vi "EMV Flow Detector.vi"(8 "error in (no error)":errorcluster, 10 "ERD Data":T1, 11 ".NET Refnum in":refnum<k24>) -> (0 "error out":errorcluster, 3 ".NET Refnum out":refnum<k24>)   [LabVIEW 2020]
uses:
  Type Definitions/GEA3 HEWH Mixing Valve.ctl
  Type Definitions/GEA3 HEWH ERD Data.ctl
  C:/TechnologyLab/NI-2010/Drivers/GEA3 Toolkit/GEA3 DLL Source/GeaCommunication.dll
  GEA3 DLL Source/GeaCommunication.dll
panel:
  in  "Detection Slope":dbl=0.5 format="%#_13g"
  out "T6 T7 Flow Dectection":bool
  out "Slope History":dbl[](array[numeric])
  out "Current T6 Temperatures Output":dbl[](array[numeric])=[75.0, 75.0, 75.0, 75.0, 75.0, 75.0, 75.0, 75.0, 75.0, 75.0, 75.0]
  out "Slope Chart T7":dbl(graph)
  out "Current T7 Temperatures":dbl[](array[numeric])
  in  "Abnormal Input Temperature":dbl=80.0
  out "Flow Detect?":bool
  in  "Entry":dbl=11.0
  in  "POLLING_TIME_MS":dbl=1000.0
  in  "FLOW_COUNTER_MAX":dbl=15.0
  in  "STARTING_TEMPERATURE":dbl=140.0
  in  "FLOW_COUNTER_THRESHOLD":dbl=1.0
  in  "T6_OFFSET_FROM_TARGET_INDICATING_FLOW":dbl=3.0
  in  "T7_DELTA_INDICATING_FLOW":dbl=10.0
  in  "T6_DELTA_INDICATING_FLOW":dbl=2.0
  in  "T7_DELTA_FLOW_THRESHOLD":dbl=0.5
  in  "T7 STOP-T6 FLOW -THRESHOLD":dbl=4.0
  out "T6 Flow Dectection":bool
  # "T6 Only"
  # "T7 Only"
  # "T6 and T7"
  # "reading now == 0\nreading in the past == 10"
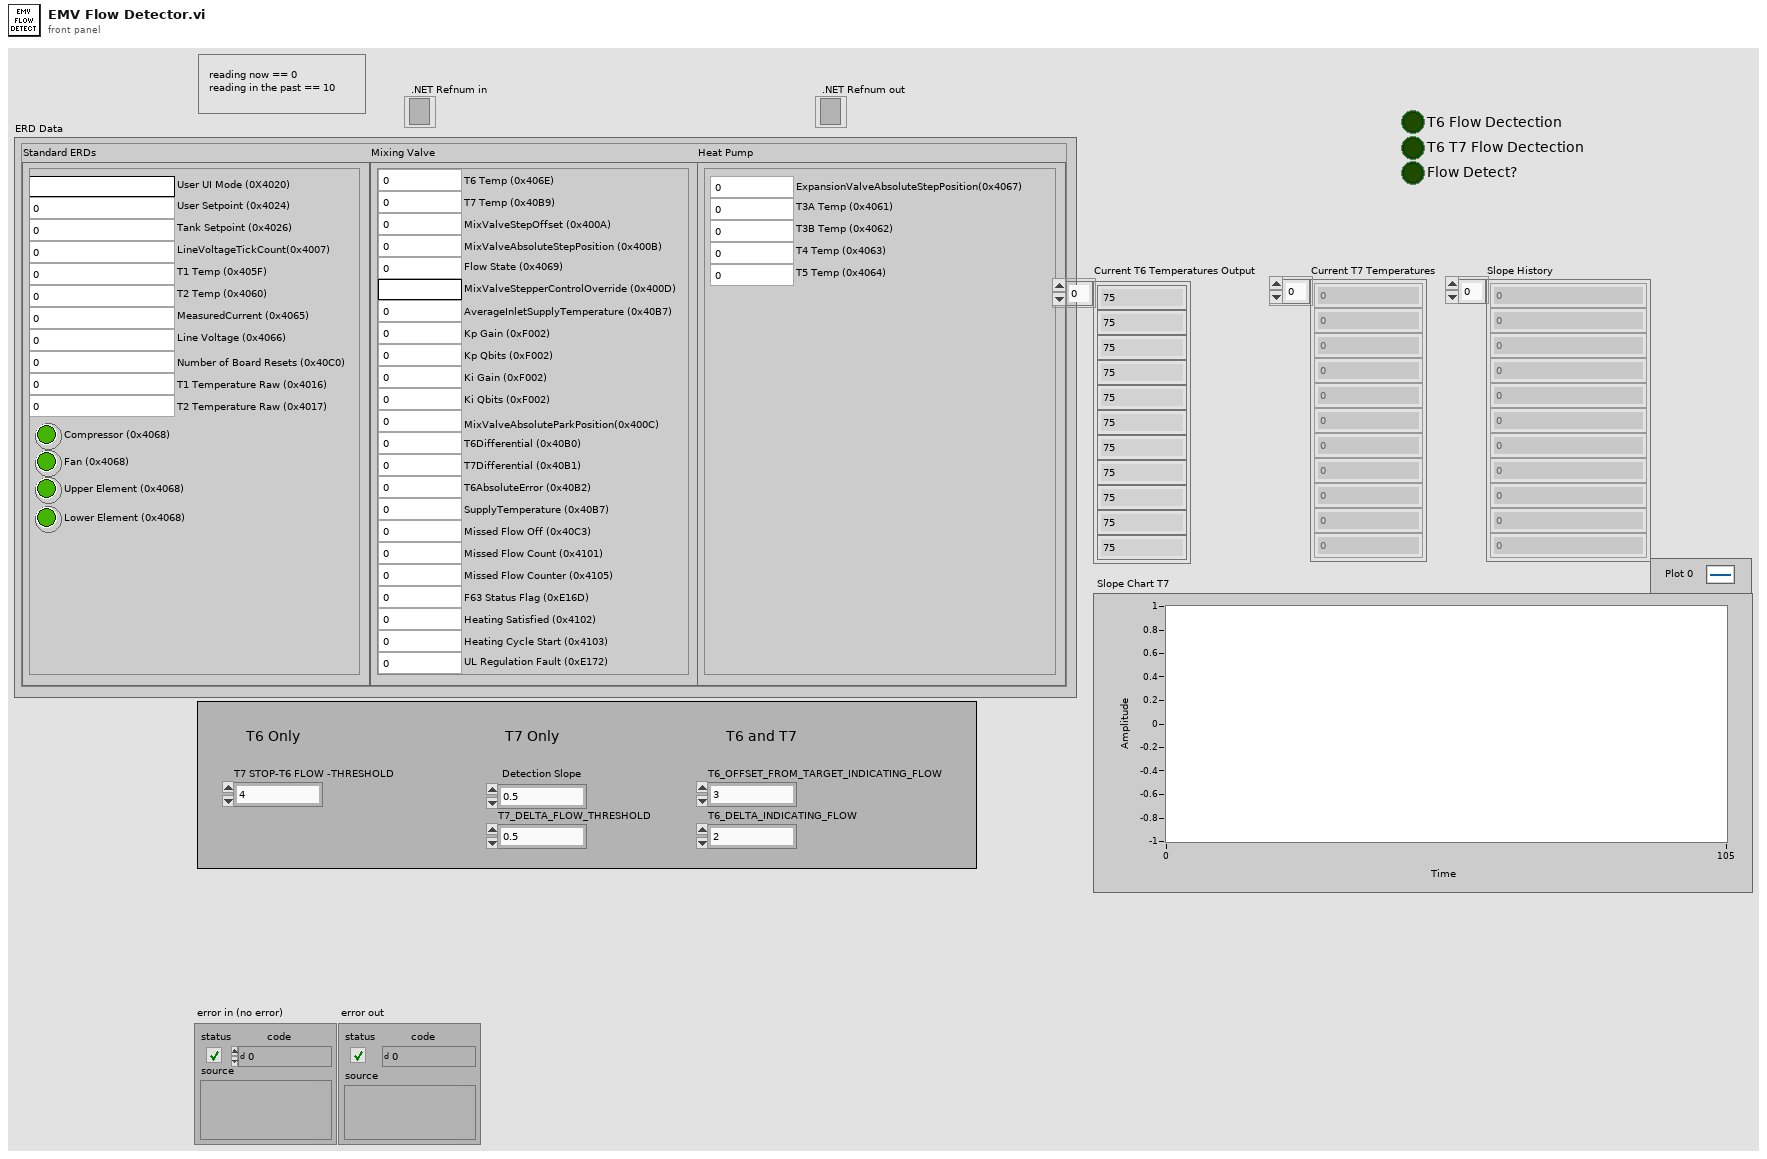
[diagram p1: front panel]
types:
  T1 = typedef "GEA3 HEWH ERD Data.ctl" = cluster{"Mixing Valve":T2, "Standard ERDs":cluster{"User UI Mode (0X4020)":string, "User Setpoint (0x4024)":u16, "Compressor (0x4068)":bool, "Lower Element (0x4068)":bool, "Upper Element (0x4068)":bool, "Fan (0x4068)":bool, "T1 Temp (0x405F)":dbl, "T2 Temp (0x4060)":dbl, "Line Voltage (0x4066)":dbl, "MeasuredCurrent (0x4065)":dbl, "LineVoltageTickCount(0x4007)":u16, "Number of Board Resets (0x40C0)":u16, "T1 Temperature Raw (0x4016)":u16, "T2 Temperature Raw (0x4017)":u16, "Tank Setpoint (0x4026)":u16}, "Heat Pump":cluster{"ExpansionValveAbsoluteStepPosition(0x4067)":i16, "T3A Temp (0x4061)":dbl, "T3B Temp (0x4062)":dbl, "T4 Temp (0x4063)":dbl, "T5 Temp (0x4064)":dbl}}
  T2 = typedef "GEA3 HEWH Mixing Valve.ctl" = cluster{"T7 Temp (0x40B9)":dbl, "MixValveStepOffset (0x400A)":i16, "MixValveAbsoluteStepPosition (0x400B)":i16, "Flow State (0x4069)":u8, "MixValveStepperControlOverride (0x400D)":string, "AverageInletSupplyTemperature (0x40B7)":dbl, "T6 Temp (0x406E)":dbl, "Kp Gain (0xF002)":u16, "Kp Qbits (0xF002)":u16, "Ki Gain (0xF002)":u16, "Ki Qbits (0xF002)":u16, "MixValveAbsoluteParkPosition(0x400C)":i16, "T7Differential (0x40B1)":dbl, "T6Differential (0x40B0)":dbl, "SupplyTemperature (0x40B7)":dbl, "Missed Flow Off (0x40C3)":u8, "T6AbsoluteError (0x40B2)":dbl, "Missed Flow Count (0x4101)":u16, "Missed Flow Counter (0x4105)":u16, "F63 Status Flag (0xE16D)":u16, "Heating Satisfied (0x4102)":u16, "Heating Cycle Start (0x4103)":u16, "UL Regulation Fault (0xE172)":u8}
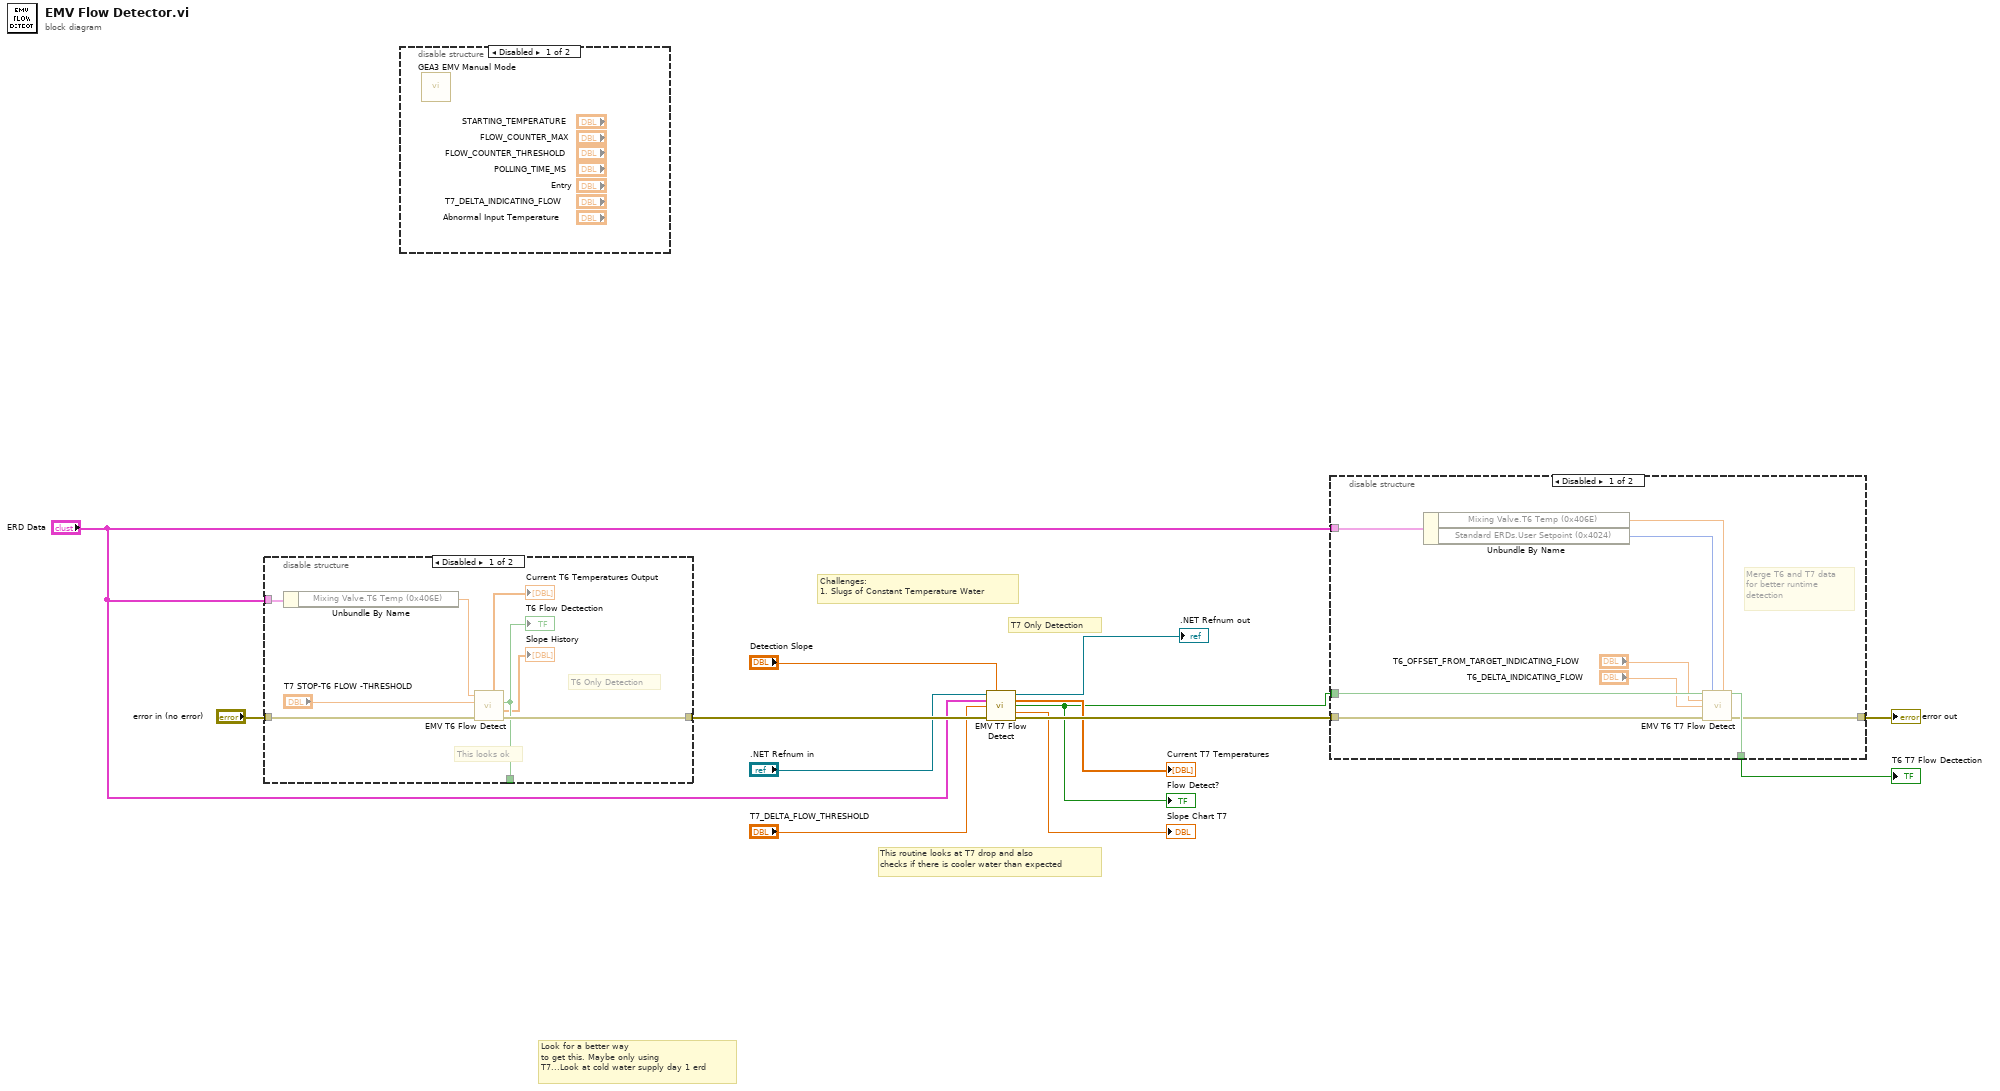
[diagram p0: block diagram]
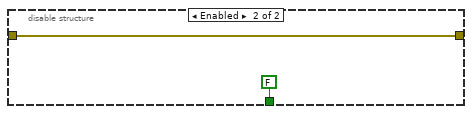
[diagram p4: hidden frame]
diagram:
  # "Challenges:\n1. Slugs of Constant Temperature Water"
  # "T7 Only Detection"
  # "Look for a better way\nto get this. Maybe only using\nT7...Look at cold water supply day 1 erd"
  # "This routine looks at T7 drop and also\nchecks if there is cooler water than expected"
  n1 = disable-structure shown="Disabled" {
    disable-tunnel: "error in (no error)" -> [w21 w23]
    disable-tunnel: [w20 w23] -> w12
    disable-tunnel: [w18 FALSE ("Flow Dectection")] -> _
    disable-tunnel: "ERD Data" -> [w15 _]
    frame Disabled {
      # "T6 Only Detection"
      # "This looks ok"
      n2 = Unbundle By Name(w15) -> ("Mixing Valve.T6 Temp (0x406E)"=w14:dbl)
      n3 = call "EMV T6 Flow Detect.vi"("error in (no error)"=w21, "T6_DELTA_FLOW_THRESHOLD"="T7 STOP-T6 FLOW -THRESHOLD", "T6 Temp"=w14) -> ("error out"=w20:errorcluster, "Slope History"=→"Slope History":dbl[], "Flow Dectection"=w18:bool, "Current T6 Temperatures Output"=→"Current T6 Temperatures Output":dbl[])  [unwired: 5 in]
      "T6 Flow Dectection" <- w18
    }
    frame Enabled {
    }
  }
  n4 = disable-structure shown="Disabled" {
    frame Disabled {
      n5 = call "GEA3 EMV Manual Mode.vi"() -> ()  [unwired: 10 in, 2 out]
    }
    frame Enabled {
    }
  }
  n6 = call "EMV T7 Flow Detect.vi"(".NET Refnum in"=".NET Refnum in", "Detection Slope"="Detection Slope", "ERD Data"="ERD Data", "T7_DELTA_FLOW_THRESHOLD"="T7_DELTA_FLOW_THRESHOLD", "error in (no error)"=w12) -> (".NET Refnum out"=→".NET Refnum out":refnum<k24>, "Current T7 Temperatures"=→"Current T7 Temperatures":dbl[], "Flow Detect?"=w2:bool, "T7 Slope Chart"=→"Slope Chart T7":dbl, "error out"=w11:errorcluster)  [unwired: 6 in]
  "Flow Detect?" <- w2
  n7 = disable-structure shown="Disabled" {
    disable-tunnel: w11 -> [w32 w33]
    disable-tunnel: [w31 _] -> w8
    disable-tunnel: [w30 w33] -> w6
    disable-tunnel: w2 -> [w29 _]
    disable-tunnel: "ERD Data" -> [w26 _]
    frame Disabled {
      # "Merge T6 and T7 data\nfor better runtime \ndetection"
      n8 = Unbundle By Name(w26) -> ("Mixing Valve.T6 Temp (0x406E)"=w25:dbl, "Standard ERDs.User Setpoint (0x4024)"=w24:u16)
      n9 = call "EMV T6 T7 Flow Detect.vi"("T7 Detect?"=w29, "User Setpoint Temperature"=w24, "Mixing Valve.T6 Temp (0x406E)"=w25, "T6_OFFSET_FROM_TARGET_INDICATING_FLOW"="T6_OFFSET_FROM_TARGET_INDICATING_FLOW", "T6_DELTA_INDICATING_FLOW"="T6_DELTA_INDICATING_FLOW", "error in (no error)"=w32) -> ("Flow Dectection"=w31:bool, "error out"=w30:errorcluster)  [unwired: 8 in]
    }
    frame Enabled {
    }
  }
  "error out" <- w6
  "T6 T7 Flow Dectection" <- w8
